vi "CONTROL CONVEYOR_2.vi"() -> ()   [LabVIEW 2018]
panel:
  in  "stop":bool
  out "Slide 2":u16(slide) scale=0.0..500.0
  in  "Slide":u16(slide) scale=0.0..10.0
  out "Pict Ring":u16(ring)
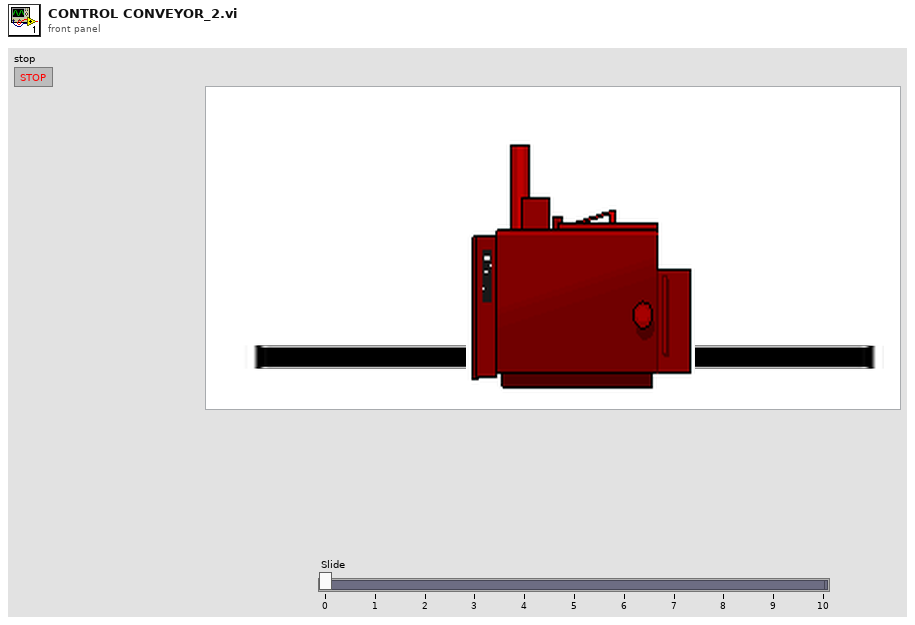
[diagram p1: front panel]
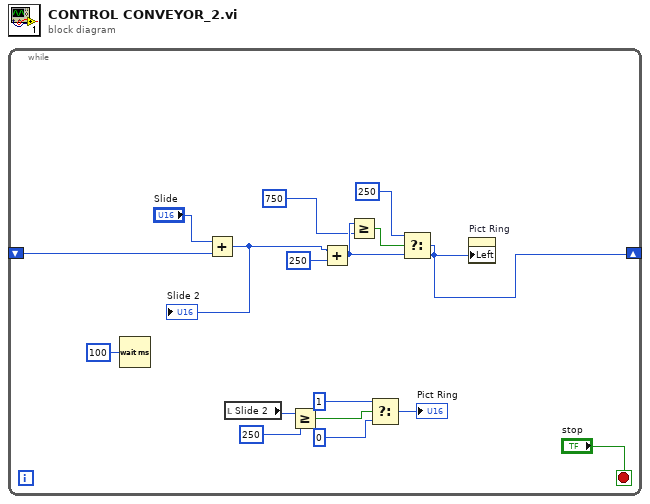
[diagram p0: block diagram]
diagram:
  n1 = while {
    shift-right: [w4] -> _
    shift-left: _ -> [w3]
    stop <- "stop" stop-if-true
    n2 = Wait (ms)(milliseconds to wait=u32 100) -> ()  [unwired: 1 out]
    n3 = Add(x="Slide", y=w3) -> (x+y=w6:u16)
    "Slide 2" <- w6
    n4 = local read "Slide 2"() -> (w14:u16)
    n5 = Greater Or Equal?(x=w14, y=u16 250) -> (x >= y?=w12:bool)
    n6 = Add(x=w6, y=u16 250) -> (x+y=w9:u16)
    n7 = Greater Or Equal?(x=w9, y=u16 750 ("t")) -> (x >= y?=w10:bool)
    n8 = Select(t=u16 1, s=w12, f=u16 0) -> (s? t:f=→"Pict Ring":u16)
    n9 = Select(t=u16 250, s=w10, f=w9) -> (s? t:f=w4:u16)
    n10 = property on="Pict Ring" class="Ring (strict)"("Left"=w4) -> ()  [unwired: 2 in, 2 out]
  }
